vi "Get FPGA Reference.vi"(8 "error in (no error)":errorcluster, 11 "nCRD in":refnum<class "nCRD.lvclass">) -> (0 "error out":errorcluster, 2 "Accessors:FPGA Ref":T1, 3 "nCRD Out":refnum<class "nCRD.lvclass">)   [LabVIEW 2015, in "nCRD.lvclass"]
uses:
  nCRD.lvclass
  FPGA Ref.ctl
  Session/Raw FPGA/FPGA Session.lvclass
  nCRD.lvclass/nCRD.ctl
  Session/Raw FPGA/FPGA Session.lvclass/FPGA Session.ctl
  Session/Raw FPGA/Read FPGA Ref.vi
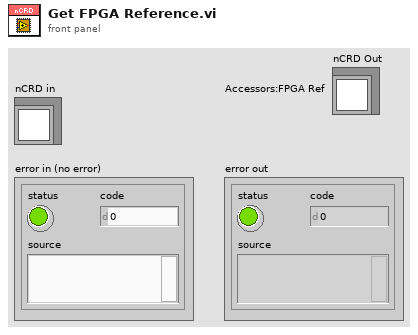
[diagram p1: front panel]
types:
  T1 = typedef "FPGA Ref.ctl" = refnum<k20>
  T2 = typedef "Session - Root.lvclass/Session Handle.ctl" = refnum<data-value>
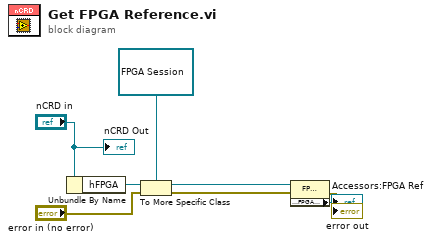
[diagram p0: block diagram]
diagram:
  n1 = Unbundle By Name("nCRD in") -> ("hFPGA"=w3:T2)
  n2 = To More Specific Class(target class=refnum<data-value> refnum ("hFPGA"), reference=w3, error in="error in (no error)") -> (specific class reference=w1:refnum<data-value>, error out=w8:errorcluster)
  n3 = property class="FPGA Session"(reference=w1, error in=w8) -> (error out=→"error out":errorcluster, "Accessors:FPGA Ref"=→"Accessors:FPGA Ref":T1)  [unwired: 1 out]
  "nCRD Out" <- "nCRD in"
